vi "Retriggerable Analog Input (STC2).vi"() -> ()   [LabVIEW 2009]
doc: "I. Description:\nThis example demonstrates how to generate a finite digital pulse train from a Counter Output Channel. And use the pulse train as the clock source for an analog input operation."
uses:
  <vilib>/DAQmx/configure/trigger.llb/DAQmx Start Trigger (Digital Edge).vi
  <vilib>/DAQmx/configure/timing.llb/DAQmx Timing (Implicit).vi
  <vilib>/DAQmx/create/channels.llb/DAQmx Create Channel (CO-Pulse Generation-Frequency).vi
  <vilib>/DAQmx/configure/timing.llb/DAQmx Timing (Sample Clock).vi
  <vilib>/DAQmx/create/channels.llb/DAQmx Create Channel (AI-Voltage-Basic).vi
  <vilib>/DAQmx/read.llb/DAQmx Read (Analog 1D DBL 1Chan NSamp).vi
  Program Files/National Instruments/LabVIEW 2009/resource/objmgr/daqmx.rc
panel:
  in  "analog input channels":tag="Dev1/ai2"
  in  "samples per channel":i32=10
  in  "stop":bool
  out "data":dbl[](graph)=[0.11633395532614343, 2.322477792337649, 2.49304052741351, 2.4512898694732237, 0.7765741109067276, -1.6028776767751645, -2.866070770695397, -2.8212456872470555, -1.0924868869830124, 1.3269366026043294]
  in  "initial delay":dbl format="%.6f"
  in  "idle state":i32(ring)=10214 items=["High"=10192, "Low"=10214]
  in  "counter":tag="Dev1/ctr0"
  in  "frequency":dbl=10.0 format="%.6f"
  in  "duty cycle":dbl=0.5 format="%.6f"
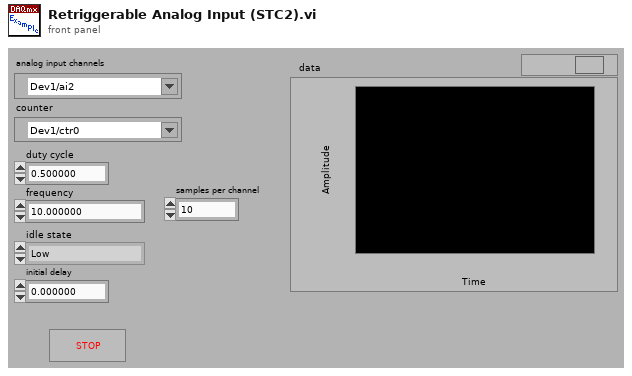
[diagram p1: front panel]
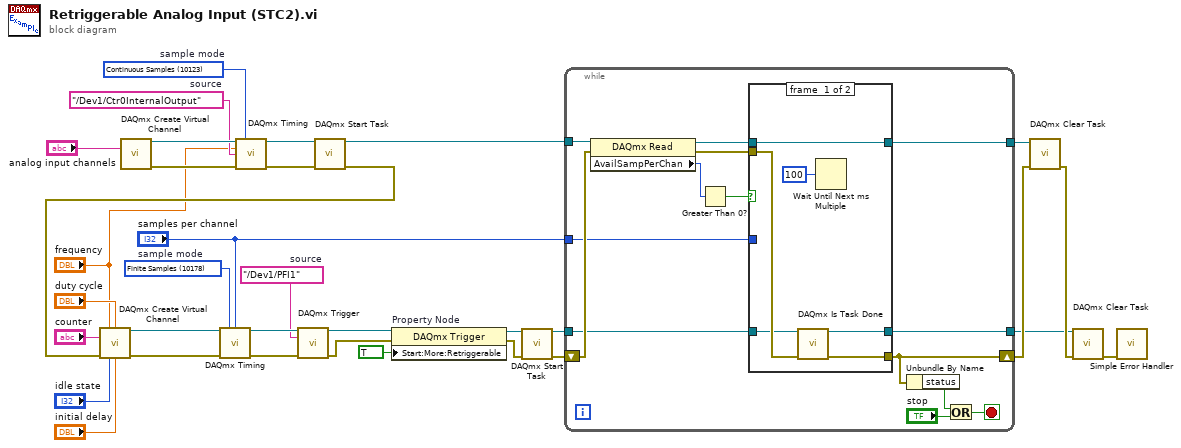
[diagram p0: block diagram]
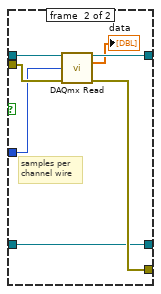
[diagram p2: hidden frame]
diagram:
  w7 = 10123 items=["Finite Samples"=10178, "Continuous Samples"=10123, "Hardware Timed Single Point"=12522]  # sample mode
  w9 = tag "/Dev1/Ctr0InternalOutput"  # source
  w21 = tag "/Dev1/PFI1"  # source
  w24 = 10178 items=["Finite Samples"=10178, "Continuous Samples"=10123]  # sample mode
  n1 = call-poly <vilib>:"DAQmx Create Virtual Channel.vi"("physical channels"="analog input channels") -> ("task out"=w15:refnum<k21>, "error out"=w12:errorcluster)  [unwired: 13 in]
  n2 = call-poly <vilib>:"DAQmx Timing.vi"("task/channels in"=w15, "sample mode"=w7, "rate"="frequency", "source"=w9, "error in"=w12) -> ("task out"=w14:refnum<k21>, "error out"=w11:errorcluster)  [unwired: 9 in]
  n3 = call <vilib>:"DAQmx Start Task.vi"("task/channels in"=w14, "error in"=w11) -> ("task out"=w13:refnum<k21>, "error out"=w10:errorcluster)  [unwired: 12 in]
  n4 = call-poly <vilib>:"DAQmx Create Virtual Channel.vi"("frequency"="frequency", "duty cycle"="duty cycle", "counter"="counter", "error in"=w10, "idle state"="idle state", "initial delay"="initial delay") -> ("task out"=w26:refnum<k21>, "error out"=w25:errorcluster)  [unwired: 8 in]
  n5 = call-poly <vilib>:"DAQmx Timing.vi"("task/channels in"=w26, "sample mode"=w24, "samples per channel"="samples per channel", "error in"=w25) -> ("task out"=w23:refnum<k21>, "error out"=w22:errorcluster)  [unwired: 10 in]
  n6 = call-poly <vilib>:"DAQmx Trigger.vi"("task/channels in"=w23, "source"=w21, "error in"=w22) -> ("task out"=w20:refnum<k21>, "error out"=w19:errorcluster)  [unwired: 11 in]
  n7 = property on="Property Node" class="DAQmx Trigger"(reference=w20, error in=w19, "Start:More:Retriggerable"=TRUE ("Start.Retriggerable")) -> (reference out=w17:refnum<k21>, error out=w16:errorcluster)
  n8 = call <vilib>:"DAQmx Start Task.vi"("task/channels in"=w17, "error in"=w16) -> ("task out"=w29:refnum<k21>, "error out"=w28:errorcluster)  [unwired: 12 in]
  n9 = while {
    tunnel: w29 -> [w37]
    tunnel: [w36] -> w3
    shift-right: [w35] -> w5
    shift-left: w28 -> [w42]
    tunnel: w13 -> [w43]
    tunnel: [w39] -> w6
    tunnel: "samples per channel" -> [w34]
    stop <- w45 stop-if-true
    n10 = property class="DAQmx Read"(reference=w43, error in=w42) -> (reference out=w40:refnum<k21>, error out=w38:errorcluster, "AvailSampPerChan"=w44:u32)
    n11 = Greater Than 0?(x=w44) -> (x > 0?=w41:bool)
    n12 = case shown="True" w41 {
      tunnel: [w52 w59] -> w39
      tunnel: w40 -> [w52 w60]
      tunnel: w38 -> [w51 w58]
      tunnel: w37 -> [w50 w56]
      tunnel: [w49 w56] -> w36
      tunnel: [w48 w57] -> w35
      tunnel: w34 -> [_ w54]
      frame #0 {
        n13 = call <vilib>:"DAQmx Is Task Done.vi"("task/channels in"=w50, "error in"=w51) -> ("task out"=w49:refnum<k21>, "error out"=w48:errorcluster)  [unwired: 11 in, 1 out]
        n14 = Wait Until Next ms Multiple(millisecond multiple=u32 100) -> ()  [unwired: 1 out]
      }
      frame #1 {
        # "samples per\nchannel wire"
        n15 = call-poly <vilib>:"DAQmx Read.vi"("task/channels in"=w60, "number of samples per channel"=w54, "error in"=w58) -> ("task out"=w59:refnum<k21>, "data"=→"data":dbl[], "error out"=w57:errorcluster)  [unwired: 10 in]
      }
    }
    n16 = Unbundle By Name "Unbundle By Name"(w35) -> ("status"=w47:bool)
    n17 = Or(x=w47, y="stop") -> (x .or. y?=w45:bool)
  }
  n18 = call <vilib>:"DAQmx Clear Task.vi"("task in"=w6, "error in"=w5) -> ("error out"=w4:errorcluster)  [unwired: 13 in]
  n19 = call <vilib>:"DAQmx Clear Task.vi"("task in"=w3, "error in"=w4) -> ("error out"=w27:errorcluster)  [unwired: 13 in]
  n20 = call <vilib>:"Simple Error Handler.vi"("error in (no error)"=w27) -> ()  [unwired: 4 in, 5 out]
